vi "generateWaveform.vi"(8 "error in (no error)":errorcluster, 11 "WaveformGenerator in":refnum<class "WaveformGenerator.lvclass">) -> (0 "error out":errorcluster, 2 "Signal Out":dbl, 3 "WaveformGenerator out":refnum<class "WaveformGenerator.lvclass">)   [LabVIEW 2015, in "WaveformGenerator.lvclass"]
uses:
  WaveformGenerator.lvclass
  WaveformGenerator.lvclass/WaveformGenerator.ctl
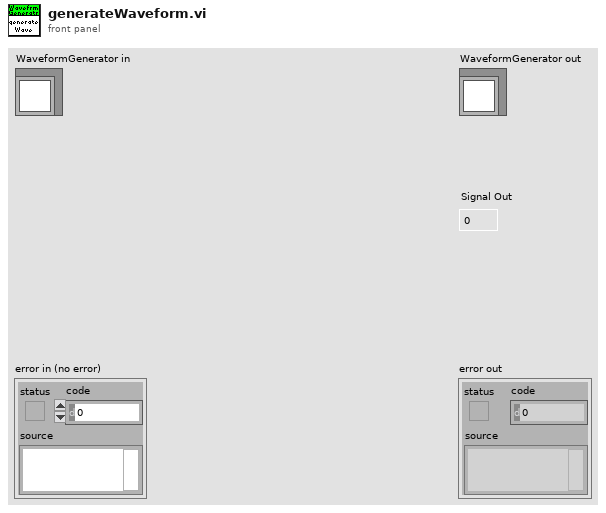
[diagram p1: front panel]
types:
  T1 = typedef "FAMTTypedefs.lvlib/Waveform.ctl" = enum16{"Sine", "Triangle", "Square", "Sawtooth", "Chirp", "Gaussian", "Trapezoid"}
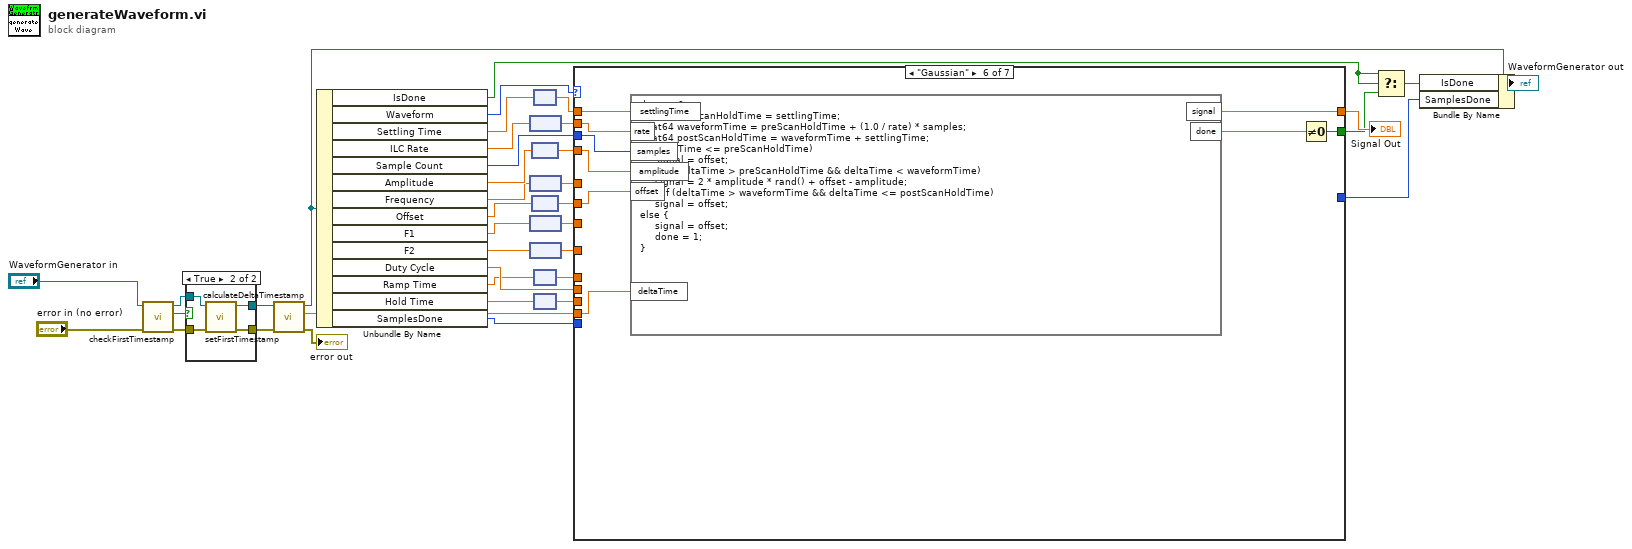
[diagram p0: block diagram]
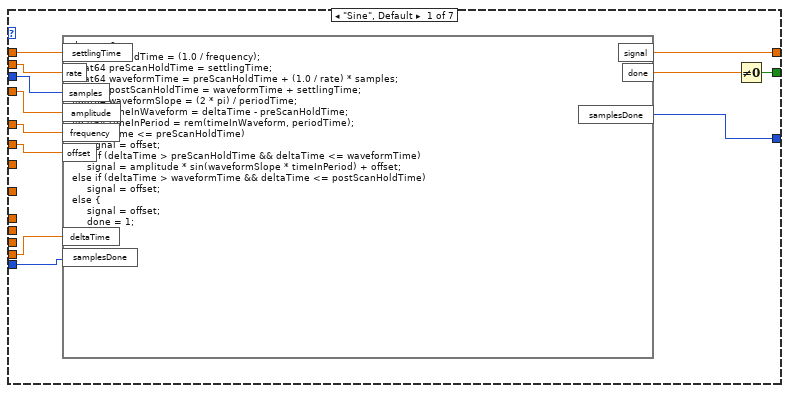
[diagram p2: hidden frame]
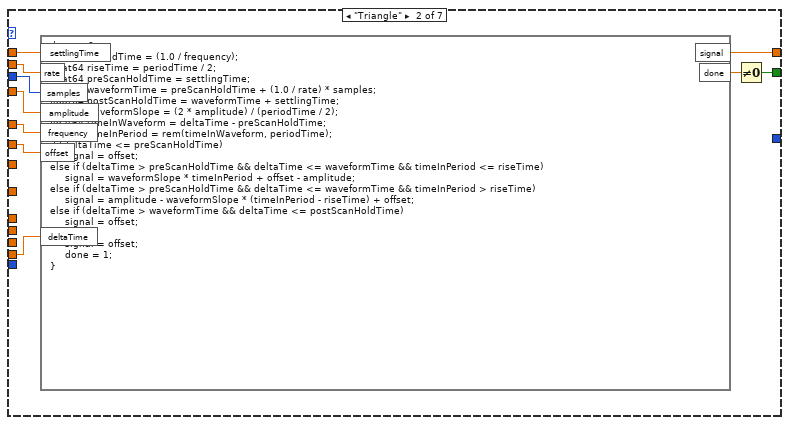
[diagram p3: hidden frame]
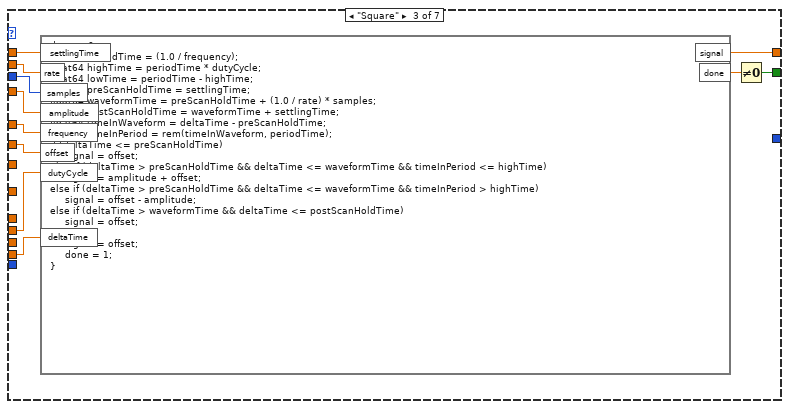
[diagram p4: hidden frame]
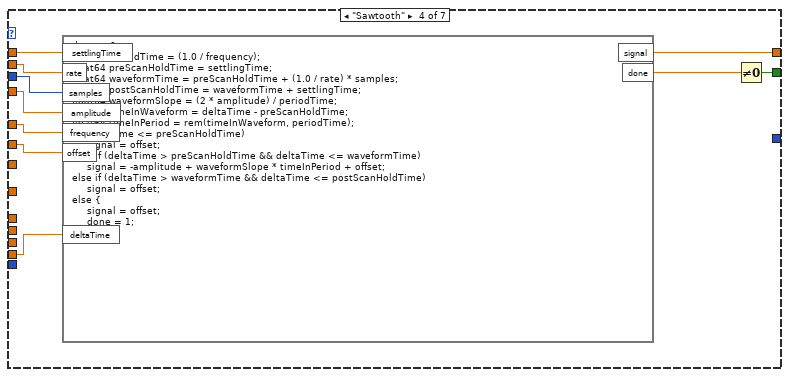
[diagram p5: hidden frame]
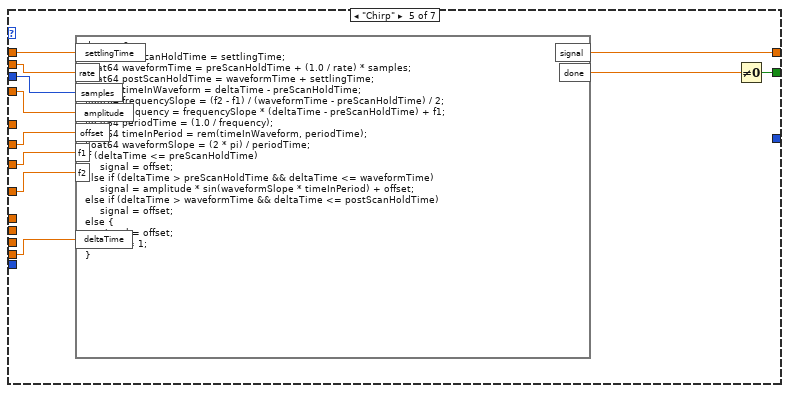
[diagram p6: hidden frame]
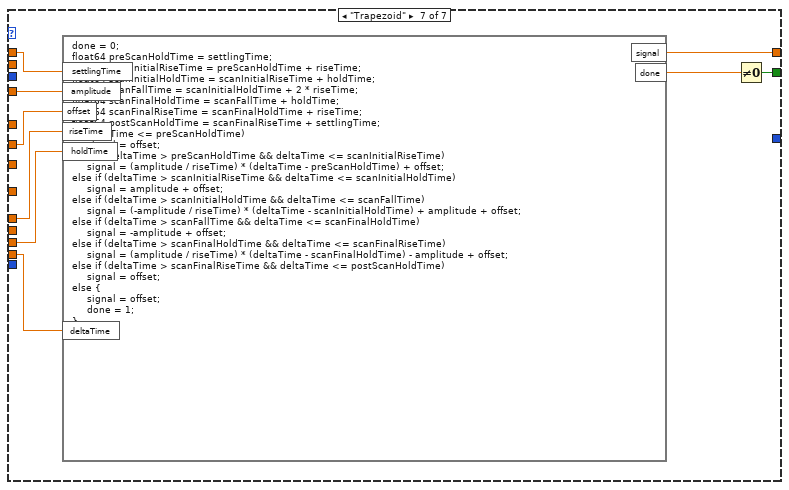
[diagram p7: hidden frame]
diagram:
  n1 = call "checkFirstTimestamp.vi"("error in (no error)"="error in (no error)", "WaveformGenerator in"="WaveformGenerator in") -> ("error out"=w36:errorcluster, "IsFirst"=w38:bool, "WaveformGenerator out"=w37:refnum<class "WaveformGenerator.lvclass">)  [unwired: 7 in]
  n2 = case shown="True" w38 {
    tunnel: w37 -> [w40 w44]
    tunnel: [w40 w43] -> w35
    tunnel: w36 -> [w39 w42]
    tunnel: [w39 w41] -> w34
    frame False {
    }
    frame True {
      n3 = call "setFirstTimestamp.vi"("error in (no error)"=w42, "WaveformGenerator in"=w44) -> ("error out"=w41:errorcluster, "WaveformGenerator out"=w43:refnum<class "WaveformGenerator.lvclass">)  [unwired: 8 in]
    }
  }
  n4 = call "calculateDeltaTimestamp.vi"("error in (no error)"=w34, "WaveformGenerator in"=w35) -> ("error out"=→"error out":errorcluster, "Delta Timestamp"=w17:dbl, "WaveformGenerator out"=w7:refnum<class "WaveformGenerator.lvclass">)  [unwired: 7 in]
  n5 = Unbundle By Name(w7) -> ("IsDone"=w4:bool, "Waveform"=w15:T1, "Settling Time"=w32:dbl[unit], "ILC Rate"=w30:dbl[unit], "Sample Count"=w29:u32, "Amplitude"=w27:dbl[unit], "Frequency"=w14:dbl[unit], "Offset"=w25:dbl[unit], "F1"=w23:dbl[unit], "F2"=w21:dbl[unit], "Duty Cycle"=w12:dbl, "Ramp Time"=w11:dbl[unit], "Hold Time"=w10:dbl[unit], "SamplesDone"=w1:u32)
  n6 = node(w30) -> (w28:dbl)
  n7 = node(w14) -> (w13:dbl)
  n8 = node(w23) -> (w22:dbl)
  n9 = node(w21) -> (w20:dbl)
  n10 = node(w27) -> (w26:dbl)
  n11 = node(w25) -> (w24:dbl)
  n12 = node(w32) -> (w31:dbl)
  n13 = node(w11) -> (w8:dbl)
  n14 = node(w10) -> (w9:dbl)
  n15 = case shown="\"Gaussian\"" w15 {
    tunnel: [w49 w66 w69 w80 w90 w102 w110] -> w33
    tunnel: w31 -> [w56 w59 w71 w87 w91 w107 w116]
    tunnel: w29 -> [w54 w61 w73 w85 w93 w105 _]
    tunnel: w28 -> [w55 w60 w72 w86 w92 w106 _]
    tunnel: w26 -> [w53 w62 w74 w84 w94 w104 w115]
    tunnel: w24 -> [w52 w64 w76 w82 w95 w99 w114]
    tunnel: w22 -> [_ _ _ _ w96 _ _]
    tunnel: w20 -> [_ _ _ _ w97 _ _]
    tunnel: w17 -> [w50 w65 w70 w81 w98 w103 w111]
    tunnel: w13 -> [w51 w63 w75 w83 _ _ _]
    tunnel: w12 -> [_ _ w77 _ _ _ _]
    tunnel: w9 -> [_ _ _ _ _ _ w113]
    tunnel: w8 -> [_ _ _ _ _ _ w112]
    tunnel: [w48 w57 w68 w78 w88 w100 w108] -> w5
    tunnel: [w46 _ _ _ _ _ _] -> w2
    tunnel: w1 -> [w45 _ _ _ _ _ _]
    frame "Sine", Default {
      n16 = formula code="done = 0;\nfloat64 periodTime = (1.0 / frequency);\nfloat64 preScanHoldTime = settlingTime;\nfloat64 waveformTime = preScanHoldTime + (1.0 / rate) * samples;\nfloat64 postScanHoldTime = waveformTime + settlingTime;\nfloat64 waveformSlope = (2 * pi) / periodTime;\nfloat64 timeInWaveform = deltaTime - preScanHoldTime;\nfloat64 timeInPeriod = rem(timeInWaveform, periodTime);\nif (deltaTime <= preScanHoldTime)\n     signal = offset;\nelse if (deltaTime > preScanHoldTime && deltaTime <= waveformTime)\n     signal = amplitude * sin(waveformSlope * timeInPeriod) + offset;\nelse if (deltaTime > waveformTime && deltaTime <= postScanHoldTime)\n     signal = offset;\nelse {\n     signal = offset;\n     done = 1;\n}"("rate"=w55, "settlingTime"=w56, "samples"=w54, "amplitude"=w53, "frequency"=w51, "offset"=w52, "deltaTime"=w50, "samplesDone"=w45) -> ("signal"=w49:dbl, "done"=w47:dbl, "samplesDone"=w46:u32)
      n17 = Not Equal To 0?(x=w47) -> (x != 0?=w48:bool)
    }
    frame "Triangle" {
      n18 = formula code="done = 0;\nfloat64 periodTime = (1.0 / frequency);\nfloat64 riseTime = periodTime / 2;\nfloat64 preScanHoldTime = settlingTime;\nfloat64 waveformTime = preScanHoldTime + (1.0 / rate) * samples;\nfloat64 postScanHoldTime = waveformTime + settlingTime;\nfloat64 waveformSlope = (2 * amplitude) / (periodTime / 2);\nfloat64 timeInWaveform = deltaTime - preScanHoldTime;\nfloat64 timeInPeriod = rem(timeInWaveform, periodTime);\nif (deltaTime <= preScanHoldTime)\n     signal = offset;\nelse if (deltaTime > preScanHoldTime && deltaTime <= waveformTime && timeInPeriod <= riseTime)\n     signal = waveformSlope * timeInPeriod + offset - amplitude;\nelse if (deltaTime > preScanHoldTime && deltaTime <= waveformTime && timeInPeriod > riseTime)\n     signal = amplitude - waveformSlope * (timeInPeriod - riseTime) + offset;\nelse if (deltaTime > waveformTime && deltaTime <= postScanHoldTime)\n     signal = offset;\nelse {\n     signal = offset;\n     done = 1;\n}"("rate"=w60, "settlingTime"=w59, "samples"=w61, "amplitude"=w62, "frequency"=w63, "offset"=w64, "deltaTime"=w65) -> ("signal"=w66:dbl, "done"=w58:dbl)
      n19 = Not Equal To 0?(x=w58) -> (x != 0?=w57:bool)
    }
    frame "Square" {
      n20 = formula code="done = 0;\nfloat64 periodTime = (1.0 / frequency);\nfloat64 highTime = periodTime * dutyCycle;\nfloat64 lowTime = periodTime - highTime;\nfloat64 preScanHoldTime = settlingTime;\nfloat64 waveformTime = preScanHoldTime + (1.0 / rate) * samples;\nfloat64 postScanHoldTime = waveformTime + settlingTime;\nfloat64 timeInWaveform = deltaTime - preScanHoldTime;\nfloat64 timeInPeriod = rem(timeInWaveform, periodTime);\nif (deltaTime <= preScanHoldTime)\n     signal = offset;\nelse if (deltaTime > preScanHoldTime && deltaTime <= waveformTime && timeInPeriod <= highTime)\n     signal = amplitude + offset;\nelse if (deltaTime > preScanHoldTime && deltaTime <= waveformTime && timeInPeriod > highTime)\n     signal = offset - amplitude;\nelse if (deltaTime > waveformTime && deltaTime <= postScanHoldTime)\n     signal = offset;\nelse {\n     signal = offset;\n     done = 1;\n}"("rate"=w72, "settlingTime"=w71, "samples"=w73, "amplitude"=w74, "frequency"=w75, "offset"=w76, "deltaTime"=w70, "dutyCycle"=w77) -> ("signal"=w69:dbl, "done"=w67:dbl)
      n21 = Not Equal To 0?(x=w67) -> (x != 0?=w68:bool)
    }
    frame "Sawtooth" {
      n22 = formula code="done = 0;\nfloat64 periodTime = (1.0 / frequency);\nfloat64 preScanHoldTime = settlingTime;\nfloat64 waveformTime = preScanHoldTime + (1.0 / rate) * samples;\nfloat64 postScanHoldTime = waveformTime + settlingTime;\nfloat64 waveformSlope = (2 * amplitude) / periodTime;\nfloat64 timeInWaveform = deltaTime - preScanHoldTime;\nfloat64 timeInPeriod = rem(timeInWaveform, periodTime);\nif (deltaTime <= preScanHoldTime)\n     signal = offset;\nelse if (deltaTime > preScanHoldTime && deltaTime <= waveformTime)\n     signal = -amplitude + waveformSlope * timeInPeriod + offset;\nelse if (deltaTime > waveformTime && deltaTime <= postScanHoldTime)\n     signal = offset;\nelse {\n     signal = offset;\n     done = 1;\n}"("rate"=w86, "settlingTime"=w87, "samples"=w85, "amplitude"=w84, "frequency"=w83, "offset"=w82, "deltaTime"=w81) -> ("signal"=w80:dbl, "done"=w79:dbl)
      n23 = Not Equal To 0?(x=w79) -> (x != 0?=w78:bool)
    }
    frame "Chirp" {
      n24 = formula code="done = 0;\nfloat64 preScanHoldTime = settlingTime;\nfloat64 waveformTime = preScanHoldTime + (1.0 / rate) * samples;\nfloat64 postScanHoldTime = waveformTime + settlingTime;\nfloat64 timeInWaveform = deltaTime - preScanHoldTime;\nfloat64 frequencySlope = (f2 - f1) / (waveformTime - preScanHoldTime) / 2;\nfloat64 frequency = frequencySlope * (deltaTime - preScanHoldTime) + f1;\nfloat64 periodTime = (1.0 / frequency);\nfloat64 timeInPeriod = rem(timeInWaveform, periodTime);\nfloat64 waveformSlope = (2 * pi) / periodTime;\nif (deltaTime <= preScanHoldTime)\n     signal = offset;\nelse if (deltaTime > preScanHoldTime && deltaTime <= waveformTime)\n     signal = amplitude * sin(waveformSlope * timeInPeriod) + offset;\nelse if (deltaTime > waveformTime && deltaTime <= postScanHoldTime)\n     signal = offset;\nelse {\n     signal = offset;\n     done = 1;\n}"("rate"=w92, "settlingTime"=w91, "samples"=w93, "amplitude"=w94, "offset"=w95, "deltaTime"=w98, "f1"=w96, "f2"=w97) -> ("signal"=w90:dbl, "done"=w89:dbl)
      n25 = Not Equal To 0?(x=w89) -> (x != 0?=w88:bool)
    }
    frame "Gaussian" {
      n26 = formula code="done = 0;\nfloat64 preScanHoldTime = settlingTime;\nfloat64 waveformTime = preScanHoldTime + (1.0 / rate) * samples;\nfloat64 postScanHoldTime = waveformTime + settlingTime;\nif (deltaTime <= preScanHoldTime)\n     signal = offset;\nelse if (deltaTime > preScanHoldTime && deltaTime < waveformTime)\n     signal = 2 * amplitude * rand() + offset - amplitude;\nelse if (deltaTime > waveformTime && deltaTime <= postScanHoldTime)\n     signal = offset;\nelse {\n     signal = offset;\n     done = 1;\n}"("settlingTime"=w107, "amplitude"=w104, "offset"=w99, "deltaTime"=w103, "rate"=w106, "samples"=w105) -> ("signal"=w102:dbl, "done"=w101:dbl)
      n27 = Not Equal To 0?(x=w101) -> (x != 0?=w100:bool)
    }
    frame "Trapezoid" {
      n28 = formula code="done = 0;\nfloat64 preScanHoldTime = settlingTime;\nfloat64 scanInitialRiseTime = preScanHoldTime + riseTime;\nfloat64 scanInitialHoldTime = scanInitialRiseTime + holdTime;\nfloat64 scanFallTime = scanInitialHoldTime + 2 * riseTime;\nfloat64 scanFinalHoldTime = scanFallTime + holdTime;\nfloat64 scanFinalRiseTime = scanFinalHoldTime + riseTime;\nfloat64 postScanHoldTime = scanFinalRiseTime + settlingTime;\nif (deltaTime <= preScanHoldTime)\n     signal = offset;\nelse if (deltaTime > preScanHoldTime && deltaTime <= scanInitialRiseTime)\n     signal = (amplitude / riseTime) * (deltaTime - preScanHoldTime) + offset;\nelse if (deltaTime > scanInitialRiseTime && deltaTime <= scanInitialHoldTime)\n     signal = amplitude + offset;\nelse if (deltaTime > scanInitialHoldTime && deltaTime <= scanFallTime)\n     signal = (-amplitude / riseTime) * (deltaTime - scanInitialHoldTime) + amplitude + offset;\nelse if (deltaTime > scanFallTime && deltaTime <= scanFinalHoldTime)\n     signal = -amplitude + offset;\nelse if (deltaTime > scanFinalHoldTime && deltaTime <= scanFinalRiseTime)\n     signal = (amplitude / riseTime) * (deltaTime - scanFinalHoldTime) - amplitude + offset;\nelse if (deltaTime > scanFinalRiseTime && deltaTime <= postScanHoldTime)\n     signal = offset;\nelse {\n     signal = offset;\n     done = 1;\n}"("deltaTime"=w111, "riseTime"=w112, "holdTime"=w113, "amplitude"=w115, "offset"=w114, "settlingTime"=w116) -> ("signal"=w110:dbl, "done"=w109:dbl)
      n29 = Not Equal To 0?(x=w109) -> (x != 0?=w108:bool)
    }
  }
  "Signal Out" <- w33
  n30 = Select(t=w4, s=w4, f=w5) -> (s? t:f=w3:bool)
  n31 = Bundle By Name(cluster=w7, "IsDone"=w3, "SamplesDone"=w2) -> (→"WaveformGenerator out":refnum<class "WaveformGenerator.lvclass">)
